vi "qTNR.vi"(0 "System no.":i32=1 min=1 max=4 step=1, 5 "error in":errorcluster) -> (14 "Number of Rec. tables":i32, 19 "error out":errorcluster)   [LabVIEW 2020]
doc: "Returns the number of recording tables. \n\nC-887, F-206, M-8X0: Only for GCS syntax version = GCS 2.0 or higher (check with CSV?.vi. If CSV?.vi is not supported, syntax version is GCS 1.0)."
panel:
  # "Returns the number of recording tables."
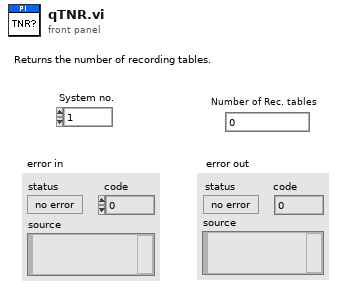
[diagram p1: front panel]
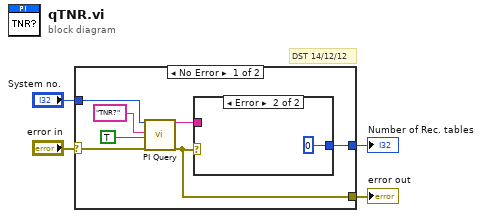
[diagram p0: block diagram]
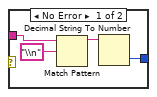
[diagram p2: hidden frame]
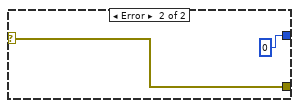
[diagram p3: hidden frame]
diagram:
  # "DST 14/12/12"
  n1 = case shown="No Error" "error in" {
    selector: "error in" -> [w5 w17]
    tunnel: [w11 0] -> w4
    tunnel: "System no." -> [w9 _]
    tunnel: [w6 w17] -> w2
    frame No Error {
      n2 = call "PI Query.vi"("System no."=w9, "String to send"="TNR?", "Attach termination char.?"=TRUE ("Attach Linefeed?"), "error in"=w5) -> ("String read"=w7:string, "error out"=w6:errorcluster)  [unwired: 3 in, 11 out]
      n3 = case shown="Error" w6 {
        tunnel: w7 -> [w14 _]
        tunnel: [w15 0] -> w11
        frame No Error {
          n4 = Match Pattern(string=w14, regular expression="\\n") -> (before substring=w12:string)  [unwired: 4 out]
          n5 = Decimal String To Number(string=w12) -> (number=w15:i32)  [unwired: 3 out]
        }
        frame Error {
        }
      }
    }
    frame Error {
    }
  }
  "error out" <- w2
  "Number of Rec. tables" <- w4
